vi "Calculate Average Center.vi"(10 "Boolean":bool, 11 "Gantry Fiducials":dbl[](array[numeric])) -> (3 "XYZTheta":dbl[](array[numeric]))   [LabVIEW 2016, in "Component Tray.lvclass"]
uses:
  Component Tray.lvclass
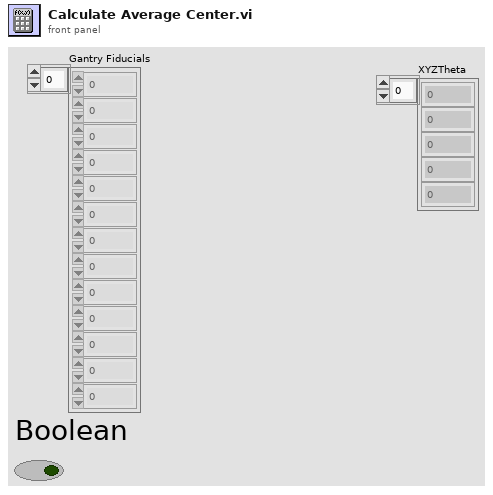
[diagram p1: front panel]
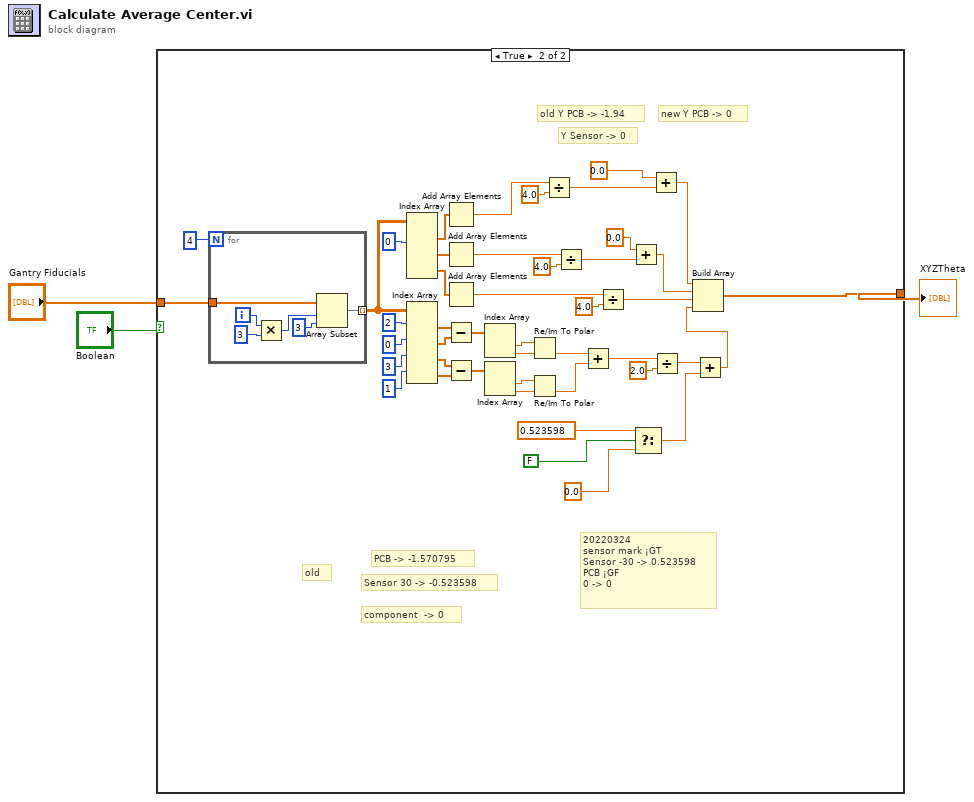
[diagram p0: block diagram]
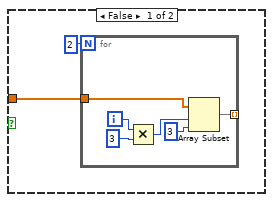
[diagram p2: hidden frame]
diagram:
  n1 = case shown="True" "Boolean" {
    tunnel: "Gantry Fiducials" -> [w4 w28]
    tunnel: [_ w22] -> w1
    frame False {
      n2 = for {
        N: 2 -> [_]
        tunnel: [w7] -> _ mode=indexing
        tunnel: w4 -> [w6]
        i -> [w11]
        n3 = Multiply(x=w11, y=3) -> (x*y=w9:i32)
        n4 = Array Subset(array=w6, index=w9, length=3) -> (w7:dbl[])
      }
    }
    frame True {
      # "20220324\nsensor mark ¡GT  \nSensor -30 -> 0.523598\nPCB ¡GF\n0 -> 0"
      # "new Y PCB -> 0"
      # "old"
      # "component  -> 0"
      # "Y Sensor -> 0"
      # "old Y PCB -> -1.94"
      # "Sensor 30 -> -0.523598"
      # "PCB -> -1.570795"
      n5 = for {
        N: 4 -> [_]
        tunnel: w28 -> [w58]
        tunnel: [w57] -> w27 mode=indexing
        i -> [w62]
        n6 = Multiply(x=w62, y=3) -> (x*y=w60:i32)
        n7 = Array Subset(array=w58, index=w60, length=3) -> (w57:dbl[])
      }
      n8 = Index Array(array=w27, index (col) #1=0 ("disabled index (col)")) -> (element #1=w55:dbl[], element #2=w54:dbl[], element #3=w25:dbl[])  [unwired: 5 in]
      n9 = Index Array(array=w27, index (row) #1=2 ("index (row)"), index (row) #2=0 ("index (row)"), index (row) #3=3 ("index (row)"), index (row) #4=1 ("index (row)")) -> (element #1=w39:dbl[], element #2=w38:dbl[], element #3=w37:dbl[], element #4=w36:dbl[])  [unwired: 4 in]
      n10 = Add Array Elements(numeric array=w55) -> (sum=w53:dbl)
      n11 = Add Array Elements(numeric array=w54) -> (sum=w52:dbl)
      n12 = Add Array Elements(numeric array=w25) -> (sum=w30:dbl)
      n13 = Subtract(x=w39, y=w38) -> (x-y=w49:dbl[])
      n14 = Subtract(x=w37, y=w36) -> (x-y=w48:dbl[])
      n15 = Index Array(array=w49) -> (element #1=w47:dbl, element #2=w46:dbl)  [unwired: 2 in]
      n16 = Index Array(array=w48) -> (element #1=w45:dbl, element #2=w44:dbl)  [unwired: 2 in]
      n17 = Re/Im To Polar(2:w46, 3:w47) -> (0:w43:dbl)  [unwired: 1 out]
      n18 = Re/Im To Polar(2:w44, 3:w45) -> (0:w42:dbl)  [unwired: 1 out]
      n19 = Divide(x=w53, y=4.0) -> (x/y=w21:dbl)
      n20 = Divide(x=w52, y=4.0) -> (x/y=w17:dbl)
      n21 = Add(x=w43, y=w42) -> (x+y=w41:dbl)
      n22 = Divide(x=w30, y=4.0) -> (x/y=w29:dbl)
      n23 = Add(x=0.0, y=w17) -> (x+y=w16:dbl)
      n24 = Select(t=0.523598 ("y"), s=FALSE, f=0.0) -> (s? t:f=w15:dbl)
      n25 = Add(x=0.0, y=w21) -> (x+y=w20:dbl)
      n26 = Divide(x=w41, y=2.0) -> (x/y=w24:dbl)
      n27 = Add(x=w24, y=w15) -> (x+y=w23:dbl)
      n28 = Build Array(w20, w16, w29, w23) -> (w22:dbl[])
    }
  }
  "XYZTheta" <- w1
